vi "Exemple_Preprocessing_KernelCenterer.vi"() -> ()   [LabVIEW 2020]
uses:
  Objet/6 - Datasets Transformation/6.3 - Processing Data/KernelCenterer/KernelCenterer.lvclass
panel:
  in  "y":string[][](array[string])
  in  "X":string[][](array[string])=[["9", "2", "-2"], ["2", "14", "-13"], ["-2", "-13", "31"]]
  out "Data":T1
  out "error out":errorcluster
  in  "error in":errorcluster caption="entrée d'erreur"
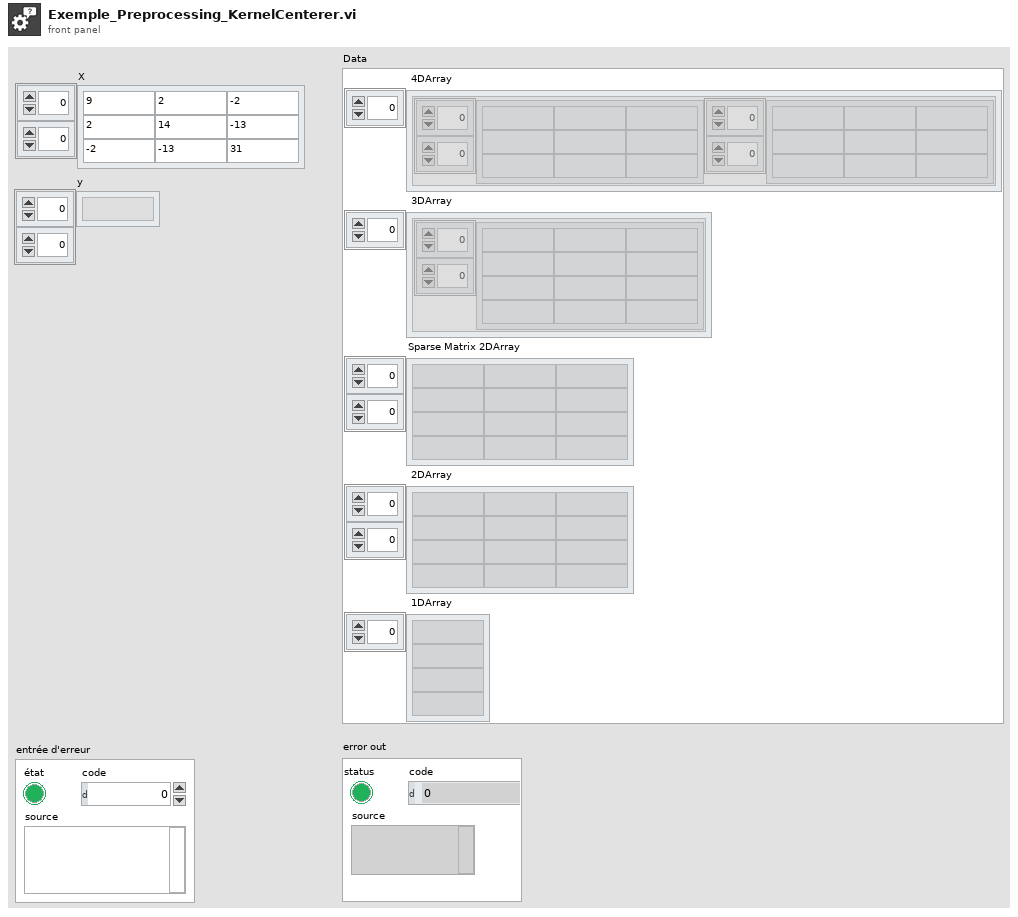
[diagram p1: front panel]
types:
  T1 = cluster{" 4DArray":cluster{"1":string[][], "2":string[][]}[], " 3DArray":cluster{"Tableau":string[][]}[], "Sparse Matrix 2DArray":string[][], " 2DArray":string[][], " 1DArray":string[]}
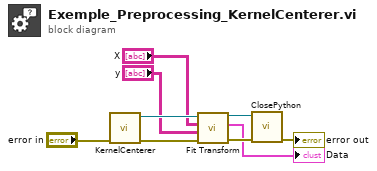
[diagram p0: block diagram]
diagram:
  n1 = call "KernelCenterer.vi"("error in (no error)"="error in") -> ("error out"=w5:errorcluster, "KernelCenterer.lvclass"=w8:refnum<class "KernelCenterer.lvclass">)  [unwired: 9 in]
  n2 = call-dynamic "Fit Transform.vi"("error in (no error)"=w5, "y"="y", "X"="X", "KernelCenterer.lvclass"=w8) -> ("error out"=w6:errorcluster, "Data"=→"Data":T1, "KernelCenterer.lvclass"=w7:refnum<class "KernelCenterer.lvclass">)  [unwired: 5 in]
  n3 = call-dynamic "ClosePython.vi"("error in (no error)"=w6, "Scikit-learn en entrée"=w7) -> ("error out"=→"error out":errorcluster)  [unwired: 8 in, 1 out]
